vi "PRL Read Buffer with Timestamp Input.vi"(7 "Time Stamp In":timestamp, 10 "Get All Signals":bool, 11 "Get Full Buffer":bool) -> (0 "Digital Signals":bool[][](array[boolean]), 1 "Analog Signals":sgl[][](array[numeric]), 2 "Phasor Signals":csg[][](array[numeric]), 3 "Timestamp":timestamp[](array[timestamp]), 4 "Has Data":bool, 5 "Time Stamp Out":timestamp, 6 "First Buffer Filled":bool)   [LabVIEW 2018, in "S3DK.lvlib" / "PMU Recorder Light.lvlib"]
doc: "Reads the newest data from the PRL Accsess Buffer."
uses:
  PMU Recorder Light.lvlib
panel:
  out "error out":errorcluster
  in  "error in (no error)":errorcluster
  # "INPUT"
  # "INTERMEDIATE"
  # "OUTPUT"
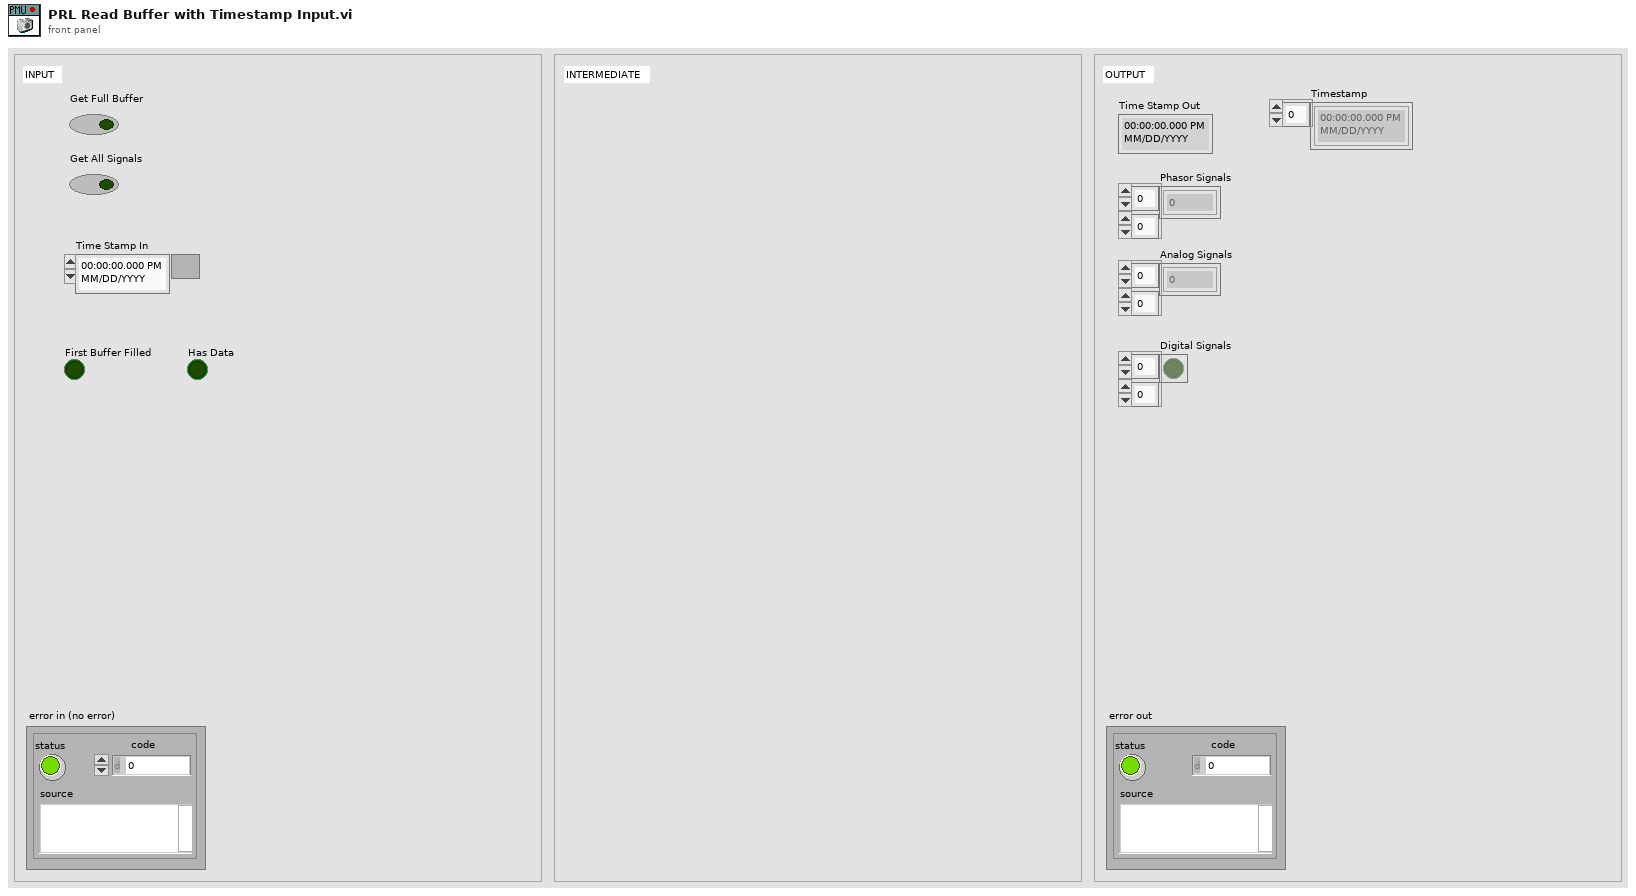
[diagram p1: front panel]
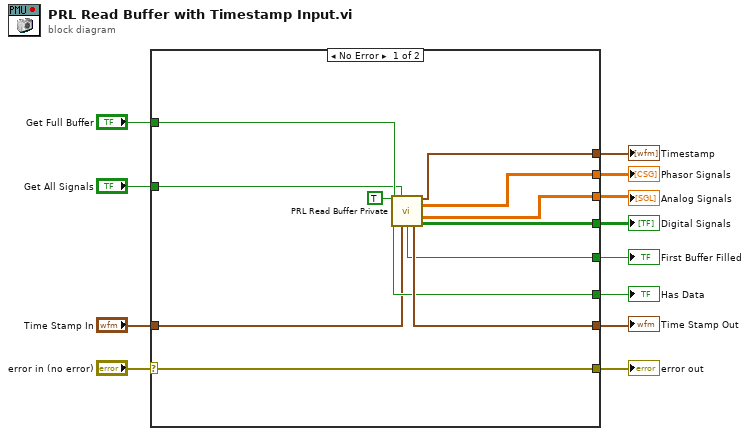
[diagram p0: block diagram]
diagram:
  n1 = case shown="No Error" "error in (no error)" {
    selector: "error in (no error)" -> [w13 w25]
    tunnel: "Get Full Buffer" -> [w24 _]
    tunnel: "Get All Signals" -> [w23 _]
    tunnel: [w22 _] -> w10
    tunnel: [w20 _] -> w9
    tunnel: [w19 _] -> w8
    tunnel: [w18 _] -> w7
    tunnel: [w17 _] -> w6
    tunnel: [w16 _] -> w5
    tunnel: [w15 _] -> w4
    tunnel: "Time Stamp In" -> [w14 _]
    tunnel: [w13 w25] -> w1
    frame No Error {
      n2 = call "PRL Read Buffer Private.vi"("Read"=TRUE, "Get All Signals"=w23, "Get Full Buffer?"=w24, "Time  Stamp In"=w14) -> ("Timestamp"=w20:timestamp[], "Phasor Signals"=w19:csg[][], "Analog Signals"=w18:sgl[][], "Has Data?"=w16:bool, "First Buffer Filled"=w15:bool, "Time Stamp Out"=w22:timestamp, "Digital Signals"=w17:bool[][])  [unwired: 4 in, 1 out]
    }
    frame Error {
    }
  }
  "Timestamp" <- w9
  "Phasor Signals" <- w8
  "Analog Signals" <- w7
  "Digital Signals" <- w6
  "Has Data" <- w5
  "First Buffer Filled" <- w4
  "Time Stamp Out" <- w10
  "error out" <- w1
